vi "dlw_Timer.vi"(6 "Worker Alias":string="Message Pump", 7 "Caller in":refnum<class "Worker.lvclass">, 8 "error in":errorcluster, 11 "Timer In":refnum<class "Timer.lvclass">) -> (0 "error out":errorcluster, 3 "Timer Out":refnum<class "Timer.lvclass">, 5 "dup Caller out":refnum<class "Worker.lvclass">)   [LabVIEW 2021, in "Timer.lvclass"]
doc: "This VI dynamically loads the Worker that owns this VI as a subWorker into <b>Caller</b>, and returns the Worker's object containing the Worker's Public Properties. Initialization data that is to be received by this Worker's <Initialize> MHL case can be wired to <b>Initialization Data</b>. The dynamically loaded Worker requires an alias ( <b>Worker Alias</b> ) which must be unique to the Worker it is called from. If a currently loaded subWorker exists with the same Alias, an error will be returned.\n\n<b>Note:</b> This VI can only be called from <b>within</b> another Worker. To call this Worker from an external LabVIEW application, load this Worker with an Asynchronous Launcher VI.\n---"
uses:
  Timer.lvclass
  <vilib>/addons/_Workers/Library/Classes/Worker/Worker.lvclass
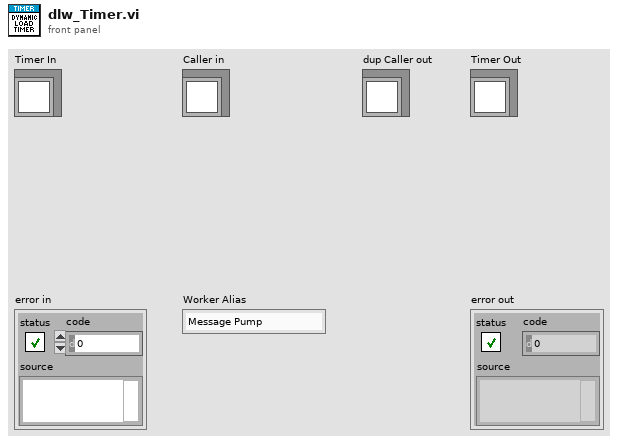
[diagram p1: front panel]
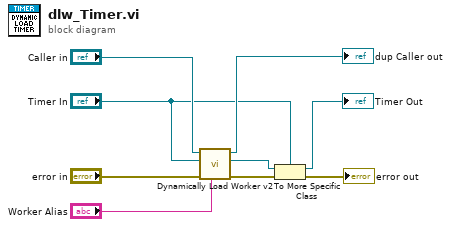
[diagram p0: block diagram]
diagram:
  n1 = call <vilib>:"Dynamically Load Worker v2.vi"("Worker Alias"="Worker Alias", "error in"="error in", "Worker to Dynamically Load"="Timer In", "Worker"="Caller in") -> ("error out"=w8:errorcluster, "Dynamically Loaded Worker out"=w3:refnum<class "Worker.lvclass">, "dup Worker out"=→"dup Caller out":refnum<class "Worker.lvclass">)  [unwired: 5 in]
  n2 = To More Specific Class(target class="Timer In", reference=w3, error in=w8) -> (specific class reference=→"Timer Out":refnum<class "Timer.lvclass">, error out=→"error out":errorcluster)
